vi "GetGradientSearchNamesAndAxes.vi"(0 "System no.":i32=1 min=1 max=4 step=1, 5 "error in":errorcluster) -> (14 "Scan Name, Scan Axis, Step Axis":string[][](array[string]), 19 "error out":errorcluster)   [LabVIEW 2020]
doc: "This VI reads all gradient search routine definitions from controller and shows names and axes in a 2D string array."
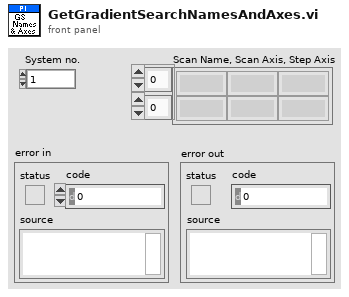
[diagram p1: front panel]
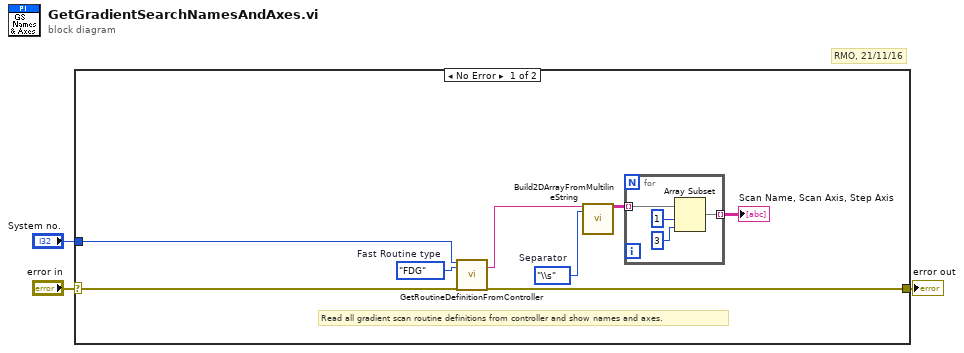
[diagram p0: block diagram]
diagram:
  # "RMO, 21/11/16"
  n1 = case shown="No Error" "error in" {
    selector: "error in" -> [w10 w16]
    tunnel: [w9 w16] -> w3
    tunnel: "System no." -> [w6 _]
    frame No Error {
      w5 = enum16{"FDG", "FDR"}."FDG"  # Fast Routine type
      w11 = enum16{"\\s", "\\t"}."\\s"  # Separator
      # "Read all gradient scan routine definitions from controller and show names and axes."
      n2 = call "GetRoutineDefinitionFromController.vi"("System no."=w6, "Fast Routine type"=w5, "error in"=w10) -> ("Routine Definitons"=w4:string, "error out"=w9:errorcluster)  [unwired: 15 out]
      n3 = call "Build2DArrayFromMultilineString.vi"("String"=w4, "Separator"=w11) -> ("2D Array out"=w7:string[][])  [unwired: 17 out]
      n4 = for {
        tunnel: w7 -> [w15] mode=indexing
        tunnel: [w12] -> w8 mode=indexing
        n5 = Array Subset(array=w15, index=1, length=3) -> (w12:string[])
      }
      "Scan Name, Scan Axis, Step Axis" <- w8
    }
    frame Error {
    }
  }
  "error out" <- w3
